vi "Pratik3-Case2-Merve Polat.vi"(1 "Dalga Frekansı(Hz)":dbl=40.0 min=40.0 step=1000000.0 format="%#_9g", 2 "Dalga Fazı(’C)":dbl min=0.0 max=360.0 step=1.0, 3 "Dalga Genliği(mV)":dbl min=0.0 max=376000.0 step=11.5, 4 "Dalga Şekli":enum16{"Kare", "Üçgen", "Sinüs", "Testere Dişi"}(ring)) -> (0 "MESSAGE":string)   [LabVIEW 2024]
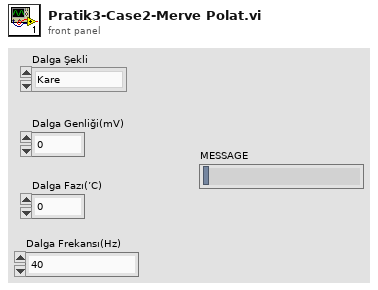
[diagram p1: front panel]
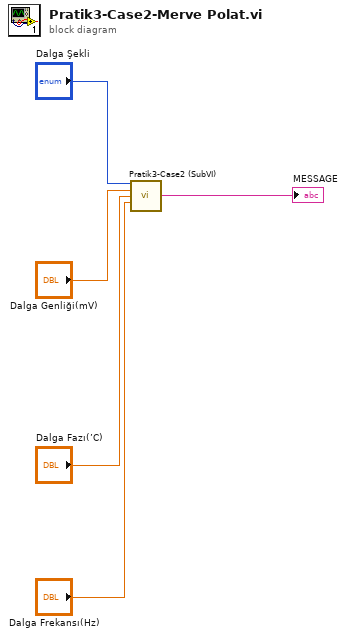
[diagram p0: block diagram]
diagram:
  n1 = call "Pratik3-Case2 (SubVI).vi"("Dalga Şekli"="Dalga Şekli", "Dalga Genliği(mV)"="Dalga Genliği(mV)", "Dalga Fazı(’C)"="Dalga Fazı(’C)", "Dalga Frekansı(Hz)"="Dalga Frekansı(Hz)") -> ("MESSAGE"=→"MESSAGE":string)  [unwired: 11 in]
